vi "测棒价值数据处理改.vi"() -> ()   [LabVIEW 2020]
uses:
  <vilib>/Utility/miscctls.llb/LVAnnotationListTypeDef.ctl
  <vilib>/Utility/miscctls.llb/LVStringsAndValuesArrayTypeDef_U16.ctl
  <vilib>/Analysis/NI_AALPro.lvlib
panel:
  out "临界段周期":dbl[](array[numeric]) caption="准临界倍增周期 (s)"
  out "临界段反应性拟合值":dbl[](array[numeric]) caption="拟合反应性 (pcm)"
  out "终端反应性均值":dbl[](array[numeric]) caption="实时反应性 (pcm)"
  out "临界段反应性均值":dbl[](array[numeric]) caption="实时反应性 (pcm)"
  out "采样间隔":dbl
  out "开始时间":timestamp
  in  "打开文件":bool
  out "历史波形图":cluster{dbl, dbl, dbl[][]}(graph)
  out "终端段点数":i32 caption="终端段点数："
  out "动态段点数":i32 caption="动态段点数："
  out "左选标时刻":timestamp caption="左选标时刻：" format="%<%.2X %x>T"
  out "临界段点数":i32 caption="临界段点数："
  out "反应性记录表":string[][](table)
  in  "刻棒选择：":u16(ring) items=["棒位"]
  in  "棒位偏移":dbl(slide) caption="棒位偏移：" min=-0.1 max=0.1 step=0.001 scale=-0.1..0.1 scale format="%#.3g"
  in  "保存表格":bool
  in  "添加记录":bool
  in  "选项卡控件":enum32{"动态段数据", "动态段曲线"}(tab)
  out "棒价值表":string[][](table) caption="动态段"
  in  "另存数据":bool
  out "价值曲线":cluster{dbl[], dbl[]}[](graph) caption="（X和Y数组）多曲线"
  out "提示信息":string="打开文件后，拖动波形图中的游标选取临界段、动态段和终端段数据进行计算。"
  out "文件信息":string
  # "临界段计算结果"
  # "终端段计算结果"
  # "坐标轴与图例"
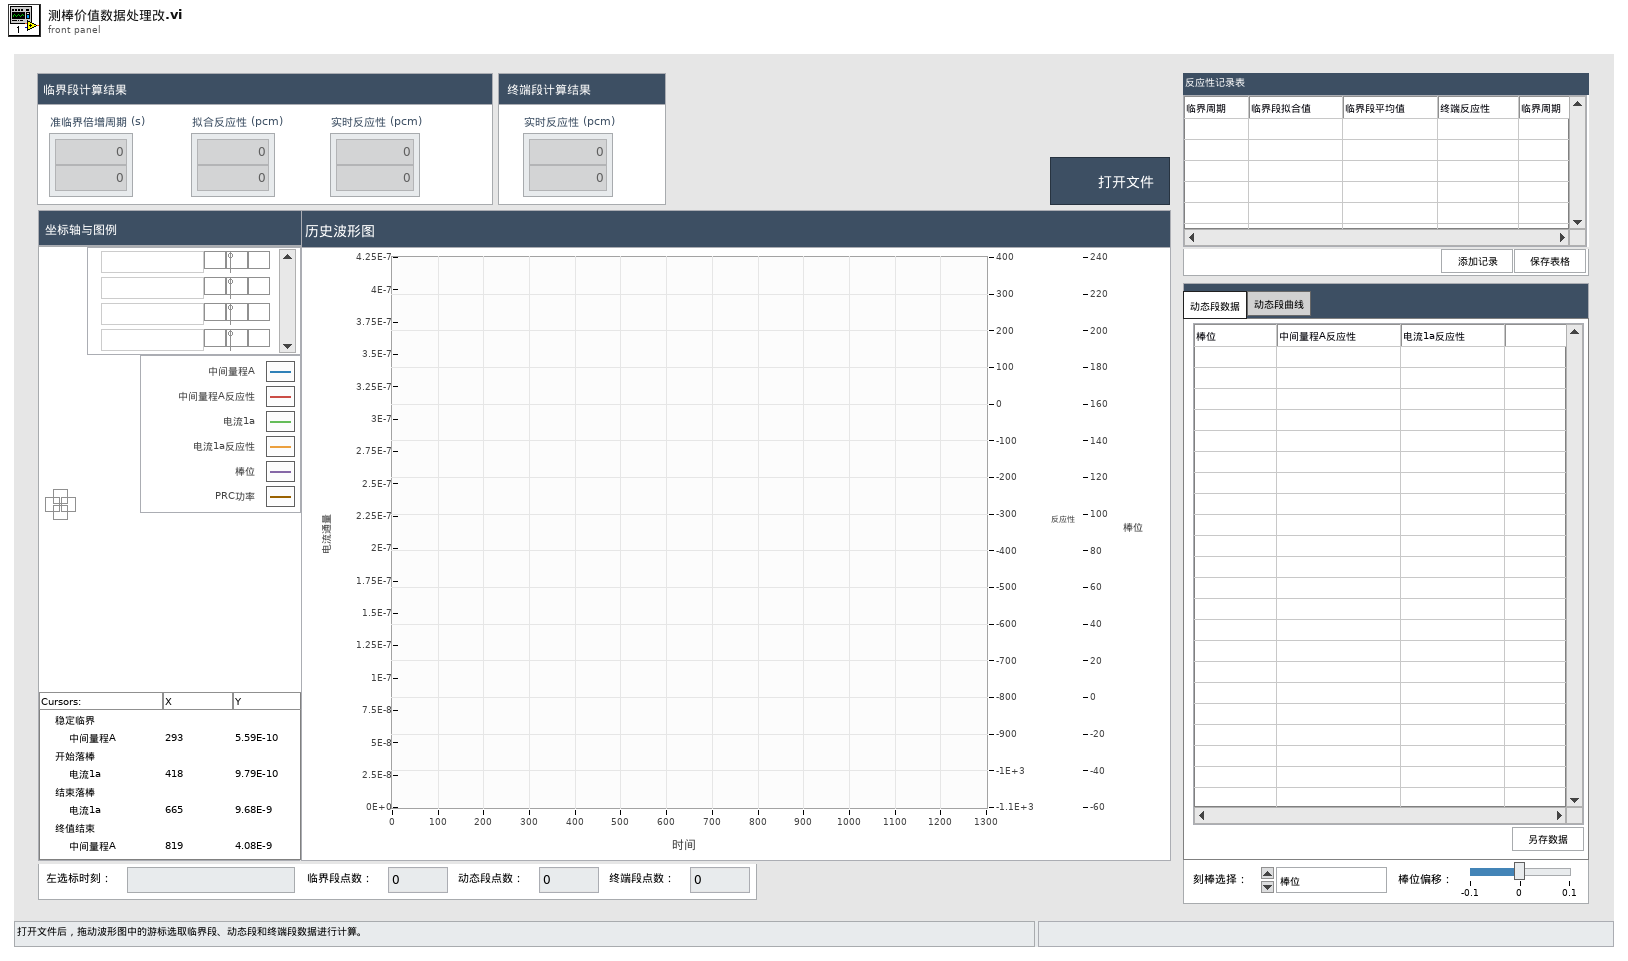
[diagram p1: front panel]
types:
  T1 = typedef "LVStringsAndValuesArrayTypeDef_U16.ctl" = cluster{"String":string, "Value":u16}[]
  T2 = typedef "LVAnnotationListTypeDef.ctl" = cluster{"Name":string, "Color":u32, "Style":u8, "Point Style":u8, "Name Visible":bool, "Allow Drag":bool, "Annotation Mode":u32, "Plot":i32, "Index":i32, "Position":cluster{"X":dbl, "Y":dbl}, "X Scale":u32, "Y Scale":u32, "Show Arrow":bool, "Lock Name":bool, "Plot Area":i32, "Label Offset":cluster{"X":dbl, "Y":dbl}}[]
  T3 = cluster{"Name":string, "Color":u32, "Style":u8, "Point Style":u8, "Name Visible":bool, "Allow Drag":bool, "Annotation Mode":u32, "Plot":i32, "Index":i32, "Position":cluster{"X":dbl, "Y":dbl}, "X Scale":u32, "Y Scale":u32, "Show Arrow":bool, "Lock Name":bool, "Plot Area":i32, "Label Offset":cluster{"X":dbl, "Y":dbl}}
  T4 = cluster{"amp min":dbl, "amp max":dbl, "damping min":dbl, "damping max":dbl, "offset min":dbl, "offset max":dbl}
  T5 = enum16{"open", "replace", "create", "open or create", "replace or create", "replace or create with confirmation"}
  T6 = typedef "LVCursorListTypeDef.ctl" = cluster{"Name":string, "Color":u32, "Style":u8, "Point Style":u8, "Name Visible":bool, "Allow Drag":bool, "Cursor Mode":u32, "Plot":i32, "Index":i32, "Position":cluster{"X":dbl, "Y":dbl}, "X Scale":u32, "Y Scale":u32, "Watch Plots":i32[], "Watch All Plots":bool, "Plot Area":i32, "Label Offset":cluster{"X":dbl, "Y":dbl}}[]
  T7 = cluster{"Name":string, "Color":u32, "Style":u8, "Point Style":u8, "Name Visible":bool, "Allow Drag":bool, "Cursor Mode":u32, "Plot":i32, "Index":i32, "Position":cluster{"X":dbl, "Y":dbl}, "X Scale":u32, "Y Scale":u32, "Watch Plots":i32[], "Watch All Plots":bool, "Plot Area":i32, "Label Offset":cluster{"X":dbl, "Y":dbl}}
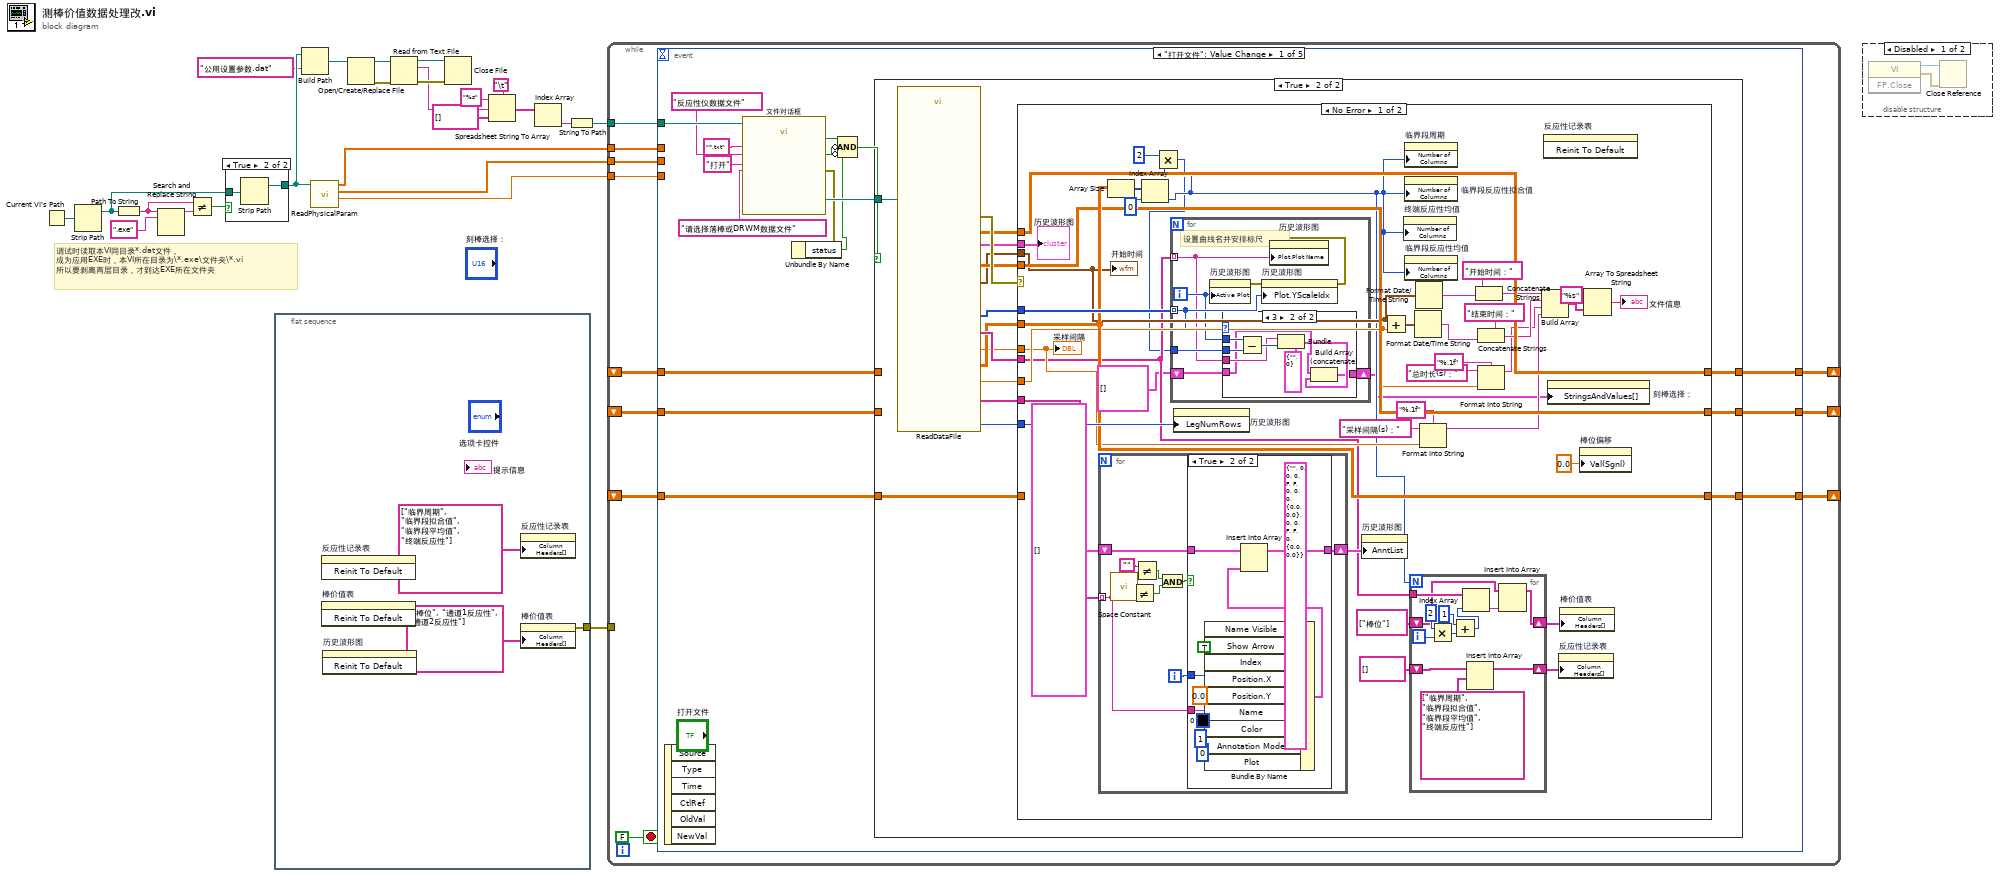
[diagram p0: block diagram]
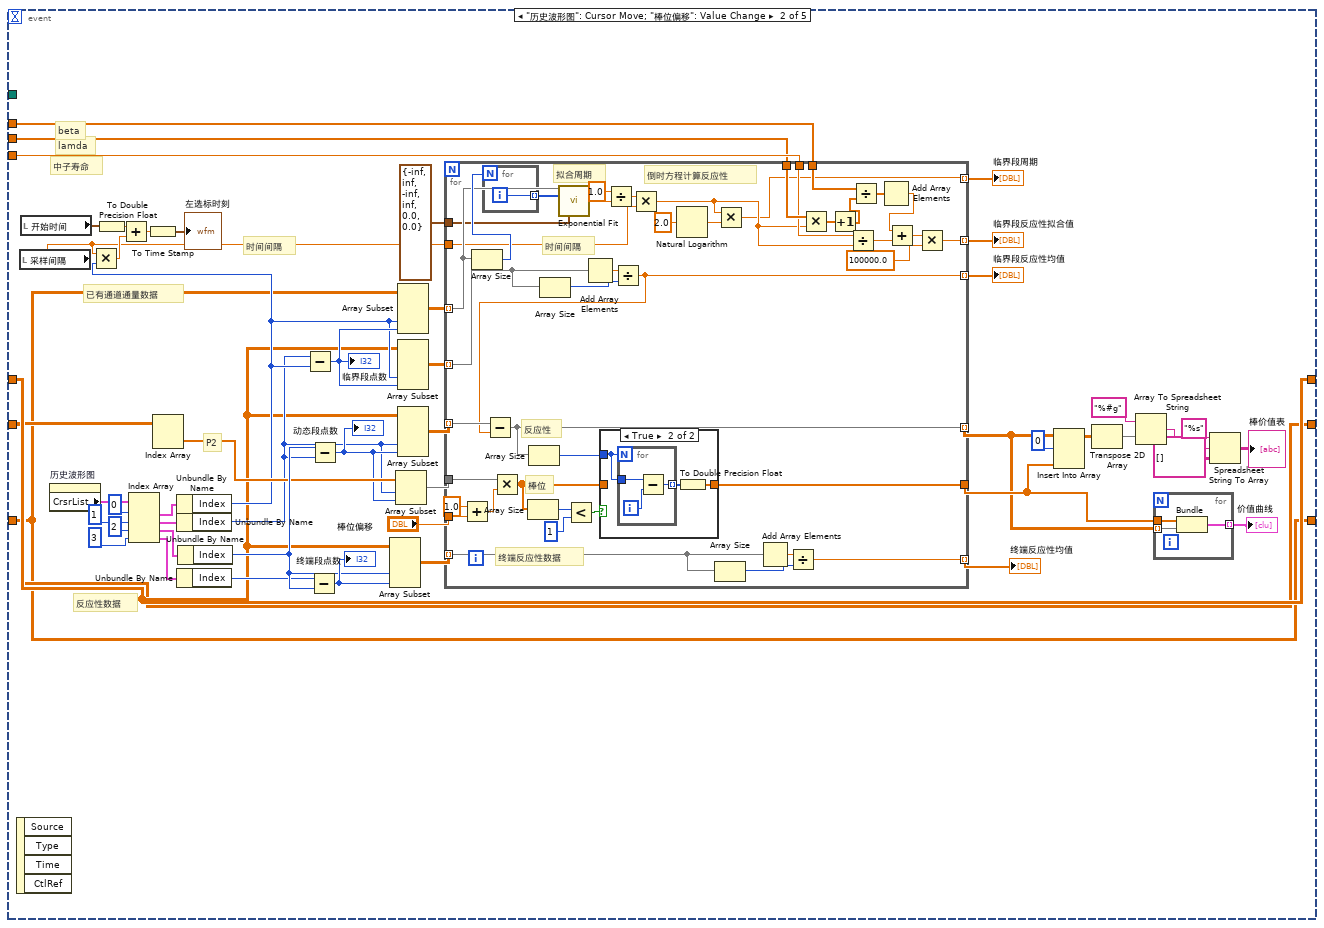
[diagram p6: hidden frame]
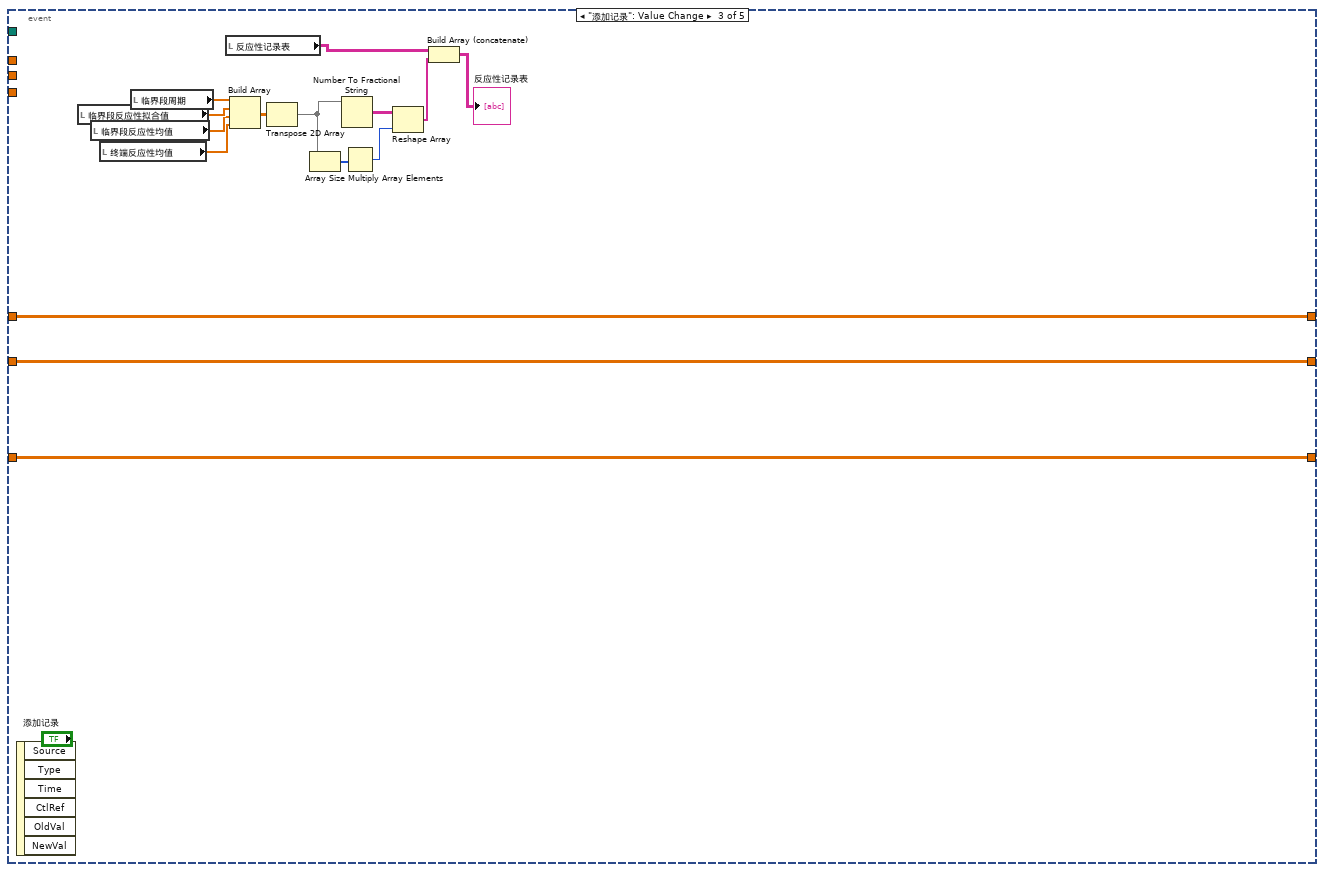
[diagram p8: hidden frame]
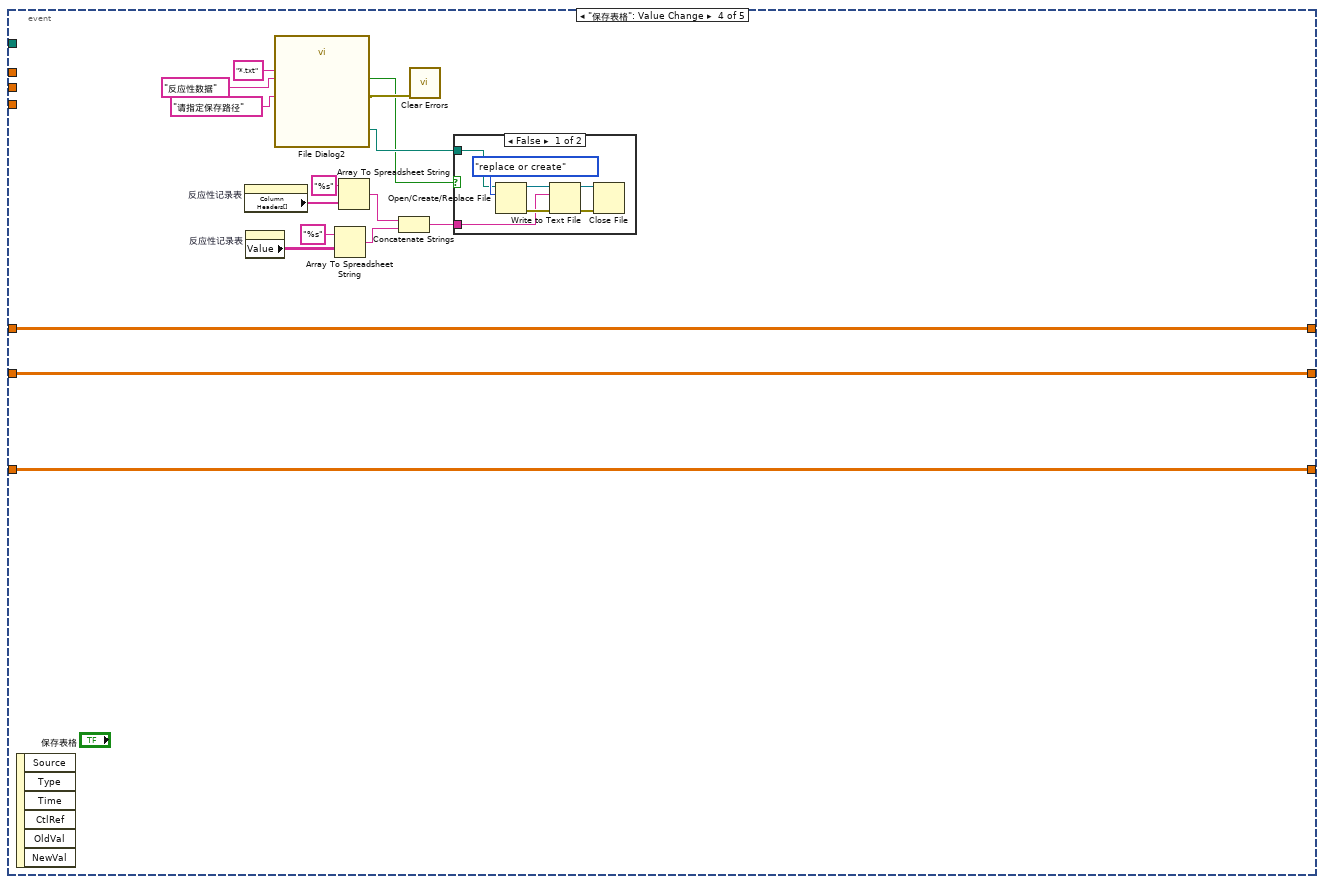
[diagram p9: hidden frame]
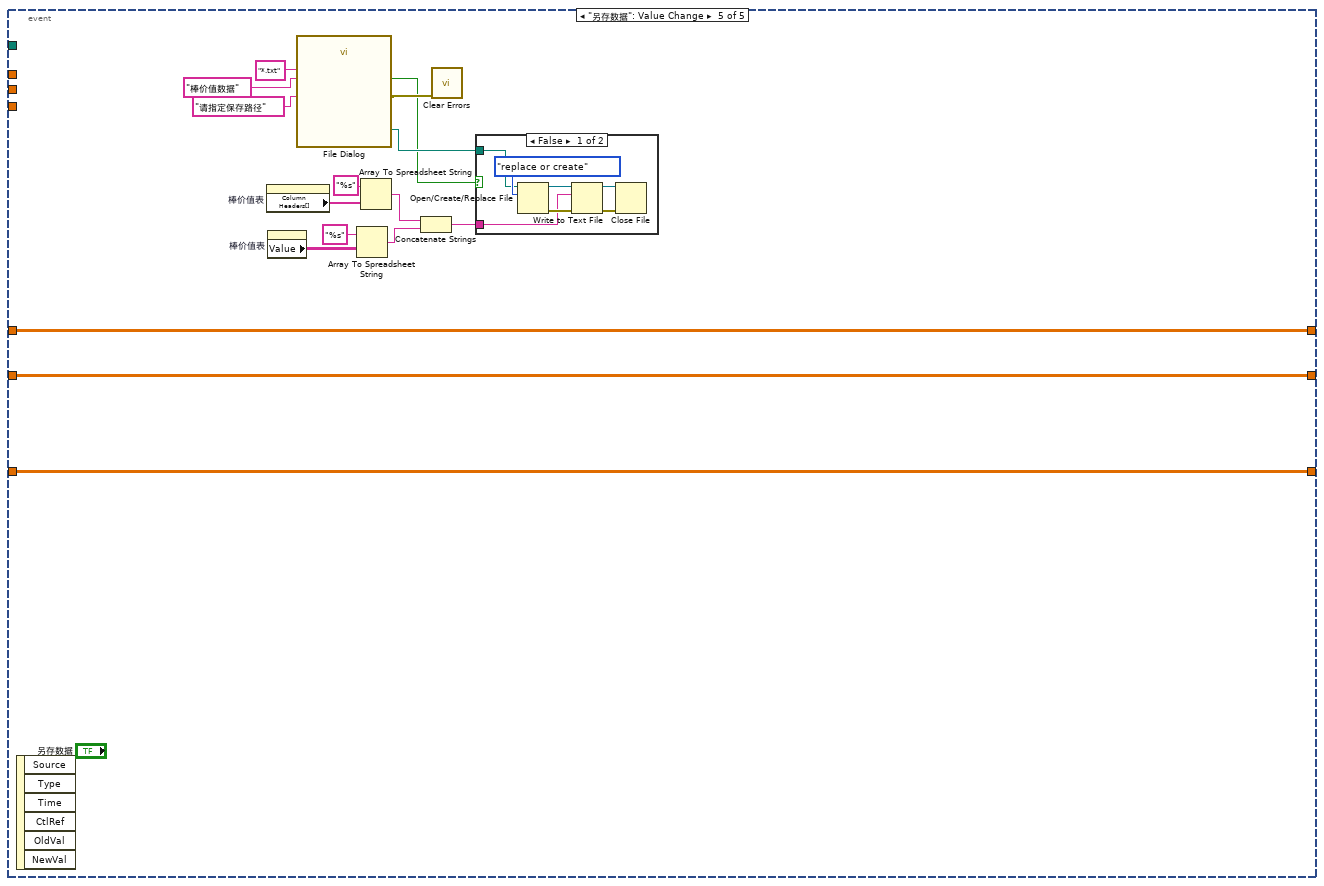
[diagram p11: hidden frame]
diagram:
  # "调试时读取本VI同目录*.dat文件，\n成为应用EXE时，本VI所在目录为\\*.exe\\文件夹\\*.vi\n所以要剥离两层目录，才到达EXE所在文件夹"
  n1 = Current VI's Path() -> (path=w19:path)
  n2 = Strip Path(path=w19) -> (stripped path=w24:path)  [unwired: 1 out]
  n3 = Path To String(path=w24) -> (string=w22:string)
  n4 = Search and Replace String(input string=w22, search string=".exe" ("搜索字符串")) -> (result string=w21:string)  [unwired: 6 in, 3 out]
  n5 = Not Equal?(x=w22, y=w21) -> (x != y?=w23:bool)
  n6 = case shown="True" w23 {
    tunnel: w24 -> [w25 w27]
    tunnel: [w25 w26] -> w18
    frame False {
    }
    frame True {
      n7 = Strip Path(path=w27) -> (stripped path=w26:path)  [unwired: 1 out]
    }
  }
  n8 = flat-sequence {
    tunnel: [w28] -> w1
    frame #0 {
      n9 = invoke on="反应性记录表" class="Tbl (strict)" method="Reinit To Default"() -> ()  [unwired: 3 in, 3 out]
      n10 = invoke on="棒价值表" class="Tbl (strict)" method="Reinit To Default"() -> ()  [unwired: 3 in, 3 out]
      n11 = invoke on="历史波形图" class="WFGraph (strict)" method="Reinit To Default"() -> ()  [unwired: 3 in, 3 out]
      n12 = property on="反应性记录表" class="Tbl (strict)"("Column Headers[]"=string[] ["临界周期", "临界段拟合值", "临界段平均值", "终端反应性"] ("行首字符串[]")) -> ()  [unwired: 2 in, 2 out]
      n13 = property on="棒价值表" class="Tbl (strict)"("Column Headers[]"=string[] ["棒位", "通道1反应性", "通道2反应性"] ("添加的数组")) -> (error out=w28:errorcluster)  [unwired: 2 in, 1 out]
    }
  }
  n14 = Build Path(base path=w18, name or relative path="公用设置参数.dat") -> (appended path=w15:path)
  n15 = call "ReadPhysicalParam.vi"("堆物理参数文件路径"=w18) -> ("中子寿命(s)"=w3:sgl, "lamda"=w2:sgl[], "beta"=w4:sgl[])  [unwired: 7 in, 1 out]
  n16 = Open/Create/Replace File(file path (use dialog)=w15) -> (refnum out=w12:refnum<file>, error out=w11:errorcluster)  [unwired: 5 in, 1 out]
  n17 = Read from Text File(file (use dialog)=w12, error in=w11) -> (refnum out=w13:refnum<file>, text=w7:string, error out=w14:errorcluster)  [unwired: 1 in, 2 out]
  n18 = Close File(refnum=w13, error in=w14) -> ()  [unwired: 2 out]
  n19 = Spreadsheet String To Array(delimiter (Tab)="\t", format string="%s", spreadsheet string=w7, array type (2D Dbl)=string[] [] ("添加的数组")) -> (array=w6:string[])
  n20 = Index Array(array=w6) -> (element=w17:string)  [unwired: 1 in]
  n21 = String To Path(string=w17) -> (path=w5:path)
  n22 = while {
    tunnel: w5 -> [w41]
    shift-right: [w39] -> _
    shift-left: _ -> [w38]
    shift-right: [w37] -> _
    shift-left: _ -> [w35]
    shift-right: [w36] -> _
    shift-left: _ -> [w34]
    tunnel: w4 -> [w33]
    tunnel: w3 -> [w32]
    tunnel: w2 -> [w31]
    tunnel: w1 -> [_]
    stop <- FALSE stop-if-true
    n23 = event shown="[0] \"打开文件\": Value Change" {
      selector: _ -> [_ _ _ _ _]
      dyn-events: _ -> [_ _ _ _ _]
      timeout: _ -> [_ _ _ _ _]
      tunnel: w41 -> [w57 _ _ _ _]
      tunnel: [w52 w175 w290 w306 w325] -> w39
      tunnel: w38 -> [w51 w175 w290 w306 w325]
      tunnel: [w50 w177 w292 w308 w327] -> w37
      tunnel: [w49 w176 w291 w307 w326] -> w36
      tunnel: w35 -> [w48 w177 w292 w308 w327]
      tunnel: w34 -> [w47 w176 w291 w307 w326]
      tunnel: w33 -> [_ w223 _ _ _]
      tunnel: w32 -> [_ w222 _ _ _]
      tunnel: w31 -> [_ w221 _ _ _]
      event "打开文件": Value Change {
        n24 = event-data() -> ()  [unwired: 1 in, 6 out]
        n25 = call "文件对话框"("start path"=w57, "prompt"="请选择落棒或DRWM数据文件", "button label"="打开", "pattern (all files)"="*.txt", "pattern label"="反应性仪数据文件") -> ("selected path"=w58:path, "exists"=w45:bool, "cancelled"=w44:bool, "error out"=w46:errorcluster)  [unwired: 7 in]
        n26 = Unbundle By Name(w46) -> ("status"=w43:bool)
        n27 = Compound Arithmetic op=AND(w45, invert w44, invert w43) -> (w42:bool)
        n28 = case shown="True" w42 {
          tunnel: w58 -> [_ w78]
          tunnel: [w61 w69] -> w52
          tunnel: w51 -> [w61 w68]
          tunnel: [w60 w65] -> w50
          tunnel: [w59 w64] -> w49
          tunnel: w48 -> [w60 _]
          tunnel: w47 -> [w59 _]
          frame False {
          }
          frame True {
            n29 = call "ReadDataFile.vi"("file path (dialog if empty)"=w78) -> ("曲线对应标尺编号"=w72:i32[], "曲线名"=w71:string[], "通量数据"=w70:dbl[][], "时间间隔"=w67:dbl, "P2数据"=w63:dbl[][], "曲线数"=w74:i32, "开始时间"=w62:timestamp, "反应性数据"=w66:dbl[][], "总时长(s)"=w75:dbl, "error out"=w77:errorcluster, "备注数组"=w73:string[], "波形簇"=w76:cluster{dbl, dbl, dbl[][]})  [unwired: 2 in, 1 out]
            n30 = case shown="No Error" w77 {
              tunnel: w76 -> [w119 _]
              tunnel: w75 -> [w98 _]
              tunnel: w74 -> [w118 _]
              tunnel: w73 -> [w115 _]
              tunnel: w72 -> [w114 _]
              tunnel: w71 -> [w84 _]
              tunnel: w70 -> [w111 _]
              tunnel: [w111 w172] -> w69
              tunnel: w68 -> [_ w172]
              tunnel: w67 -> [w96 _]
              tunnel: w66 -> [w110 w171]
              tunnel: [w110 w171] -> w65
              tunnel: [w109 w170] -> w64
              tunnel: w63 -> [w109 w170]
              tunnel: w62 -> [w103 _]
              frame No Error {
                n31 = for {
                  tunnel: w115 -> [w152] mode=indexing
                  shift-right: [w154] -> w117
                  shift-left: T2 [] ("注释列表") -> [w155]
                  i -> [w156]
                  n32 = call <vilib>:"Space Constant.vi"() -> ("String"=w157:string)
                  n33 = Not Equal?(x=w157, y=w152) -> (x != y?=w150:bool)
                  n34 = Not Equal?(x="", y=w152) -> (x != y?=w151:bool)
                  n35 = And(x=w151, y=w150) -> (x .and. y?=w149:bool)
                  n36 = case shown="True" w149 {
                    tunnel: w152 -> [_ w164]
                    tunnel: w156 -> [_ w166]
                    tunnel: w155 -> [w158 w169]
                    tunnel: [w158 w168] -> w154
                    frame False {
                    }
                    frame True {
                      w167 = TRUE ("Show Arrow")
                      n37 = Bundle By Name(cluster=T3 {"Name"="", "Color"=0, "Style"=0, "Point Style"=0, "Name Visible"=FALSE, "Allow Drag"=FALSE, "Annotation Mode"=0, "Plot"=0, "Index"=0, "Position"={"X"=0.0, "Y"=0.0}, "X Scale"=0, "Y Scale"=0, "Show Arrow"=FALSE, "Lock Name"=FALSE, "Plot Area"=0, "Label Offset"={"X"=0.0, "Y"=0.0}} ("元素"), "Name Visible"=w167, "Show Arrow"=w167, "Index"=w166, "Position.X"=w166, "Position.Y"=0.0 ("Y"), "Name"=w164, "Color"=u32 0, "Annotation Mode"=u32 1, "Plot"=0) -> (w165:T3)
                      n38 = Insert Into Array(array=w169, new element=w165) -> (w168:T2)  [unwired: 1 in]
                    }
                  }
                }
                n39 = Array Size(array=w111) -> (size(s)=w113:i32[])
                n40 = Index Array(array=w113, index=0 ("索引")) -> (element=w83:i32)
                n41 = Multiply(x=2, y=w83) -> (x*y=w81:i32)
                n42 = for {
                  tunnel: w114 -> [w137] mode=indexing
                  tunnel: w84 -> [w134] mode=indexing
                  tunnel: w81 -> [w135]
                  shift-right: [w132] -> w79
                  shift-left: T1 [] ("Strings And Values []") -> [w133]
                  i -> [w136]
                  # "设置曲线名并安排标尺"
                  n43 = property on="历史波形图" class="WFGraph (strict)"("Active Plot"=w136) -> (error out=w139:errorcluster)  [unwired: 2 in, 1 out]
                  n44 = case shown="3" w137 {
                    tunnel: w136 -> [_ w147]
                    tunnel: w135 -> [_ w148]
                    tunnel: w134 -> [_ w145]
                    tunnel: w133 -> [w140 w143]
                    tunnel: [w140 w141] -> w132
                    frame 0, Default {
                    }
                    frame 3 {
                      n45 = Subtract(x=w147, y=w148) -> (x-y=w146:i32)
                      n46 = Bundle(cluster=cluster{"String":string, "Value":u16} {"String"="", "Value"=0}, "String"=w145, "Value"=w146) -> (w142:cluster{"String":string, "Value":u16})
                      n47 = Build Array (concatenate)(w143, w142) -> (w141:T1)
                    }
                  }
                  n48 = property on="历史波形图" class="WFGraph (strict)"(error in=w139, "Plot.YScaleIdx"=w137) -> (error out=w138:errorcluster)  [unwired: 1 in, 1 out]
                  n49 = property on="历史波形图" class="WFGraph (strict)"(error in=w138, "Plot.Plot Name"=w134) -> ()  [unwired: 1 in, 2 out]
                }
                n50 = property on="历史波形图" class="WFGraph (strict)"("LegNumRows"=w118) -> ()  [unwired: 2 in, 2 out]
                n51 = property on="历史波形图" class="WFGraph (strict)"("AnntList"=w117) -> ()  [unwired: 2 in, 2 out]
                n52 = Add(x=w103, y=w98) -> (x+y=w104:timestamp)
                n53 = property on="终端反应性均值" class="Arr (strict)"("Number of Columns"=w83) -> ()  [unwired: 2 in, 2 out]
                n54 = property on="临界段周期" class="Arr (strict)"("Number of Columns"=w83) -> ()  [unwired: 2 in, 2 out]
                n55 = property on="临界段反应性拟合值" class="Arr (strict)"("Number of Columns"=w83) -> ()  [unwired: 2 in, 2 out]
                n56 = property on="临界段反应性均值" class="Arr (strict)"("Number of Columns"=w83) -> ()  [unwired: 2 in, 2 out]
                n57 = for {
                  N: w83 -> [_]
                  tunnel: w84 -> [w129]
                  shift-right: [w124] -> w108
                  shift-left: string[] ["棒位"] ("添加的数组") -> [w123]
                  shift-right: [w120] -> w105
                  shift-left: string[] [] ("行首字符串[]") -> [w121]
                  i -> [w131]
                  n58 = Multiply(x=2, y=w131) -> (x*y=w128:i32)
                  n59 = Add(x=1, y=w128) -> (x+y=w126:i32)
                  n60 = Index Array(array=w129, index=w126) -> (element=w125:string)
                  n61 = Insert Into Array(array=w121, new element=string[] ["临界周期", "临界段拟合值", "临界段平均值", "终端反应性"] ("行首字符串[]")) -> (w120:string[])  [unwired: 1 in]
                  n62 = Insert Into Array(array=w123, new element=w125) -> (w124:string[])  [unwired: 1 in]
                }
                n63 = Format Date/Time String(seconds (now)=w104) -> (date/time string=w99:string)  [unwired: 2 in]
                n64 = Format Date/Time String(seconds (now)=w103) -> (date/time string=w101:string)  [unwired: 2 in]
                n65 = Format Into String(format string="%.1f", initial string="采样间隔(s)：", w96) -> (resulting string=w89:string)  [unwired: 1 in, 1 out]
                n66 = Concatenate Strings("开始时间：" ("string"), w101) -> (w94:string)
                n67 = Concatenate Strings("结束时间：" ("string"), w99) -> (w91:string)
                n68 = Format Into String(format string="%.1f", initial string="总时长(s)：", w98) -> (resulting string=w90:string)  [unwired: 1 in, 1 out]
                n69 = Build Array(w94, w91, w90, w89) -> (w93:string[])
                n70 = invoke on="反应性记录表" class="Tbl (strict)" method="Reinit To Default"() -> ()  [unwired: 3 in, 3 out]
                n71 = property on="刻棒选择：" class="Ring (strict)"("StringsAndValues[]"=w79) -> ()  [unwired: 2 in, 2 out]
                n72 = property on="反应性记录表" class="Tbl (strict)"("Column Headers[]"=w105) -> ()  [unwired: 2 in, 2 out]
                n73 = property on="棒价值表" class="Tbl (strict)"("Column Headers[]"=w108) -> ()  [unwired: 2 in, 2 out]
                n74 = property on="棒位偏移" class="Slide (strict)"("Val(Sgnl)"=0.0 ("Value (Signaling)")) -> ()  [unwired: 2 in, 2 out]
                n75 = Array To Spreadsheet String(array=w93, 3:"%s" ("format string")) -> (spreadsheet string=→"文件信息":string)  [unwired: 1 in]
                "历史波形图" <- w119
                "开始时间" <- w103
                "采样间隔" <- w96
              }
              frame Error {
              }
            }
          }
        }
      }
      event "历史波形图": Cursor Move; "棒位偏移": Value Change {
        # "lamda"
        # "beta"
        # "中子寿命"
        # "反应性数据"
        # "P2"
        # "时间间隔"
        # "已有通道通量数据"
        n76 = event-data() -> ()  [unwired: 1 in, 4 out]
        n77 = local read "采样间隔"() -> (w173:dbl)
        n78 = local read "开始时间"() -> (w174:timestamp)
        n79 = property on="历史波形图" class="WFGraph (strict)"() -> ("CrsrList"=w216:T6)  [unwired: 2 in, 2 out]
        n80 = To Double Precision Float(number=w174) -> (double precision float=w208:dbl)
        n81 = Index Array(array=w216, index #1=0 ("index"), index #2=1 ("index"), index #3=2 ("索引"), index #4=3 ("索引")) -> (element #1=w218:T7, element #2=w220:T7, element #3=w201:T7, element #4=w200:T7)
        n82 = Index Array(array=w176) -> (element=w189:dbl[])  [unwired: 2 in]
        n83 = Unbundle By Name(w218) -> ("Index"=w180:i32)
        n84 = Multiply(x=w173, y=w180) -> (x*y=w205:dbl)
        n85 = Add(x=w208, y=w205) -> (x+y=w207:dbl)
        n86 = To Time Stamp(1:w207) -> (0:→"左选标时刻":timestamp)
        n87 = Unbundle By Name(w220) -> ("Index"=w179:i32)
        n88 = Unbundle By Name(w200) -> ("Index"=w197:i32)
        n89 = Unbundle By Name(w201) -> ("Index"=w198:i32)
        n90 = Subtract(x=w179, y=w180) -> (x-y=w213:i32)
        "临界段点数" <- w213
        n91 = Subtract(x=w197, y=w198) -> (x-y=w199:i32)
        "终端段点数" <- w199
        n92 = Subtract(x=w198, y=w179) -> (x-y=w188:i32)
        "动态段点数" <- w188
        n93 = Array Subset(array=w177, index (col)=w198, length (col)=w199) -> (w196:dbl[][])  [unwired: 2 in]
        n94 = Array Subset(array=w189, index=w179, length=w188) -> (w194:dbl[])
        n95 = Array Subset(array=w175, index (col)=w180, length (col)=w213) -> (w215:dbl[][])  [unwired: 2 in]
        n96 = Array Subset(array=w177, index (col)=w180, length (col)=w213) -> (w214:dbl[][])  [unwired: 2 in]
        n97 = Array Subset(array=w177, index (col)=w179, length (col)=w188) -> (w202:dbl[][])  [unwired: 2 in]
        n98 = for {
          tunnel: w215 -> [w254] mode=indexing
          tunnel: w222 -> [w266]
          tunnel: w223 -> [w269]
          tunnel: w221 -> [w268]
          tunnel: w214 -> [w239] mode=indexing
          tunnel: [w241] -> w211 mode=indexing
          tunnel: [w238] -> w178 mode=indexing
          tunnel: [w267] -> w212 mode=indexing
          tunnel: [w245] -> w210 mode=indexing
          tunnel: w173 -> [w247]
          tunnel: T4 {"amp min"=-inf, "amp max"=inf, "damping min"=-inf, "damping max"=inf, "offset min"=0.0, "offset max"=0.0} ("parameter bounds") -> [w249]
          tunnel: w202 -> [w240] mode=indexing
          tunnel: w196 -> [w242] mode=indexing
          tunnel: w194 -> [w237]
          tunnel: "棒位偏移" -> [w236]
          tunnel: [w229] -> w182 mode=indexing
          tunnel: [w227] -> w184
          # "棒位"
          # "反应性"
          # "终端反应性数据"
          # "时间间隔"
          # "拟合周期"
          # "倒时方程计算反应性"
          n99 = Add(x=1.0, y=w236) -> (x+y=w234:dbl)
          n100 = Array Size(array=w254) -> (size(s)=w256:i32)
          n101 = for {
            N: w256 -> [_]
            tunnel: [w277] -> w255 mode=indexing
            i -> [w277]
          }
          n102 = Multiply(x=w237, y=w234) -> (x*y=w233:dbl[])
          n103 = Array Size(array=w233) -> (size(s)=w232:i32)
          n104 = Array Size(array=w239) -> (size(s)=w257:i32)
          n105 = call <vilib>:"Exponential Fit.vi"("Y"=w254, "X"=w255, "parameter bounds"=w249) -> ("damping"=w253:dbl)  [unwired: 7 in, 5 out]
          n106 = Less?(x=w232, y=1) -> (x < y?=w230:bool)
          n107 = Add Array Elements(numeric array=w239) -> (sum=w265:dbl)
          n108 = Divide(x=1.0, y=w253) -> (x/y=w248:dbl)
          n109 = Divide(x=w265, y=w257) -> (x/y=w238:dbl)
          n110 = Subtract(x=w240, y=w238) -> (x-y=w229:dbl[])
          n111 = Array Size(array=w229) -> (size(s)=w228:i32)
          n112 = case shown="True" w230 {
            tunnel: w233 -> [w270 _]
            tunnel: w228 -> [_ w273]
            tunnel: [w270 w271] -> w227
            frame False {
            }
            frame True {
              n113 = for {
                N: w273 -> [_]
                tunnel: w273 -> [w276]
                tunnel: [w274] -> w272 mode=indexing
                i -> [w275]
                n114 = Subtract(x=w276, y=w275) -> (x-y=w274:i32)
              }
              n115 = To Double Precision Float(number=w272) -> (double precision float=w271:dbl[])
            }
          }
          n116 = Multiply(x=w248, y=w247) -> (x*y=w246:dbl)
          n117 = Natural Logarithm(1:sgl 2.0) -> (0:w250:sgl)
          n118 = Array Size(array=w242) -> (size(s)=w243:i32)
          n119 = Multiply(x=w246, y=w250) -> (x*y=w245:dbl)
          n120 = Add Array Elements(numeric array=w242) -> (sum=w244:dbl)
          n121 = Divide(x=w244, y=w243) -> (x/y=w241:dbl)
          n122 = Multiply(x=w268, y=w246) -> (x*y=w258:dbl[])
          n123 = Increment(x=w258) -> (x+1=w259:dbl[])
          n124 = Divide(x=w266, y=w246) -> (x/y=w262:dbl)
          n125 = Divide(x=w269, y=w259) -> (x/y=w264:dbl[])
          n126 = Add Array Elements(numeric array=w264) -> (sum=w263:dbl)
          n127 = Add(x=w263, y=w262) -> (x+y=w261:dbl)
          n128 = Multiply(x=w261, y=sgl 100000.0) -> (x*y=w267:dbl)
        }
        "临界段反应性均值" <- w178
        "终端反应性均值" <- w211
        "临界段反应性拟合值" <- w212
        "临界段周期" <- w210
        n129 = Insert Into Array(array=w182, index (row)=0 ("索引 (行)"), new element=w184) -> (w187:dbl[][])  [unwired: 1 in]
        n130 = Transpose 2D Array(2D array=w187) -> (transposed array=w186:dbl[][])
        n131 = Array To Spreadsheet String(array=w186, 3:"%#g" ("格式字符串")) -> (spreadsheet string=w181:string)  [unwired: 1 in]
        n132 = for {
          tunnel: w184 -> [w224]
          tunnel: w182 -> [w225] mode=indexing
          tunnel: [w226] -> w183 mode=indexing
          n133 = Bundle "Bundle"(w224, w225) -> (w226:cluster{dbl[], dbl[]})  [unwired: 1 in]
        }
        "价值曲线" <- w183
        n134 = Spreadsheet String To Array(format string="%s" ("格式字符串"), spreadsheet string=w181, array type (2D Dbl)=string[][] [] ("添加的数组")) -> (array=→"棒价值表":string[][])  [unwired: 1 in]
      }
      event "添加记录": Value Change {
        n135 = event-data() -> ()  [unwired: 1 in, 6 out]
        n136 = local read "临界段反应性拟合值"() -> (w288:dbl[])
        n137 = local read "临界段反应性均值"() -> (w287:dbl[])
        n138 = local read "终端反应性均值"() -> (w286:dbl[])
        n139 = local read "临界段周期"() -> (w289:dbl[])
        n140 = local read "反应性记录表"() -> (w284:string[][])
        n141 = Build Array(w289, w288, w287, w286) -> (w278:dbl[][])
        n142 = Transpose 2D Array(2D array=w278) -> (transposed array=w279:dbl[][])
        n143 = Array Size(array=w279) -> (size(s)=w281:i32[])
        n144 = Number To Fractional String(number=w279) -> (F-format string=w285:string[][])  [unwired: 3 in]
        n145 = Multiply Array Elements(1:w281) -> (0:w280:i32)
        n146 = Reshape Array(w285, w280) -> (w283:string[])
        n147 = Build Array (concatenate)(w284, w283) -> (→"反应性记录表":string[][])
      }
      event "保存表格": Value Change {
        n148 = event-data() -> ()  [unwired: 1 in, 6 out]
        n149 = property on="反应性记录表" class="Tbl (strict)"() -> ("Column Headers[]"=w305:string[])  [unwired: 2 in, 2 out]
        n150 = property on="反应性记录表" class="Tbl (strict)"() -> ("Value"=w302:string[][])  [unwired: 2 in, 2 out]
        n151 = call "File Dialog2"("prompt"="请指定保存路径" ("提示"), "pattern (all files)"="*.txt" ("类型（所有文件）"), "pattern label"="反应性数据" ("默认名称")) -> ("selected path"=w299:path, "cancelled"=w298:bool, "error out"=w300:errorcluster)  [unwired: 9 in, 1 out]
        n152 = Array To Spreadsheet String(array=w302, 3:"%s" ("format string")) -> (spreadsheet string=w301:string)  [unwired: 1 in]
        n153 = Array To Spreadsheet String(array=w305, 3:"%s" ("格式字符串")) -> (spreadsheet string=w304:string)  [unwired: 1 in]
        n154 = Concatenate Strings(w304, w301) -> (w303:string)
        n155 = call <vilib>:"Clear Errors.vi"("error in (no error)"=w300) -> ()  [unwired: 5 in, 2 out]
        n156 = case shown="False" w298 {
          tunnel: w303 -> [w310 _]
          tunnel: w299 -> [w309 _]
          frame False {
            n157 = Open/Create/Replace File(file path (use dialog)=w309, operation (0:open)=T5."replace or create") -> (refnum out=w313:refnum<file>, error out=w315:errorcluster)  [unwired: 4 in, 1 out]
            n158 = Write to Text File(file (use dialog)=w313, text=w310, error in=w315) -> (refnum out=w312:refnum<file>, error out=w311:errorcluster)  [unwired: 1 in, 1 out]
            n159 = Close File(refnum=w312, error in=w311) -> ()  [unwired: 2 out]
          }
          frame True {
          }
        }
      }
      event "另存数据": Value Change {
        n160 = event-data() -> ()  [unwired: 1 in, 6 out]
        n161 = property on="棒价值表" class="Tbl (strict)"() -> ("Column Headers[]"=w331:string[])  [unwired: 2 in, 2 out]
        n162 = property on="棒价值表" class="Tbl (strict)"() -> ("Value"=w324:string[][])  [unwired: 2 in, 2 out]
        n163 = call "File Dialog"("prompt"="请指定保存路径" ("提示"), "pattern (all files)"="*.txt" ("类型（所有文件）"), "pattern label"="棒价值数据" ("默认名称")) -> ("selected path"=w320:path, "cancelled"=w319:bool, "error out"=w321:errorcluster)  [unwired: 9 in, 1 out]
        n164 = Array To Spreadsheet String(array=w324, 3:"%s" ("format string")) -> (spreadsheet string=w323:string)  [unwired: 1 in]
        n165 = Array To Spreadsheet String(array=w331, 3:"%s" ("格式字符串")) -> (spreadsheet string=w329:string)  [unwired: 1 in]
        n166 = Concatenate Strings(w329, w323) -> (w328:string)
        n167 = call <vilib>:"Clear Errors.vi"("error in (no error)"=w321) -> ()  [unwired: 5 in, 2 out]
        n168 = case shown="False" w319 {
          tunnel: w328 -> [w333 _]
          tunnel: w320 -> [w332 _]
          frame False {
            n169 = Open/Create/Replace File(file path (use dialog)=w332, operation (0:open)=T5."replace or create") -> (refnum out=w336:refnum<file>, error out=w338:errorcluster)  [unwired: 4 in, 1 out]
            n170 = Write to Text File(file (use dialog)=w336, text=w333, error in=w338) -> (refnum out=w335:refnum<file>, error out=w334:errorcluster)  [unwired: 1 in, 1 out]
            n171 = Close File(refnum=w335, error in=w334) -> ()  [unwired: 2 out]
          }
          frame True {
          }
        }
      }
    }
  }
  n172 = disable-structure shown="Disabled" {
    frame Disabled {
      n173 = invoke class="VI" method="FP.Close"() -> (reference out=w340:refnum<vi>, error out=w339:errorcluster)  [unwired: 3 in, 1 out]
      n174 = Close Reference(reference=w340, error in (no error)=w339) -> ()  [unwired: 1 out]
    }
    frame Enabled {
    }
  }
